vi "MainMeasure.vi"(8 "error in (no error)":errorcluster, 11 "TestMeasureStep in":refnum<class "TestMeasureStep.lvclass">) -> (0 "error out":errorcluster, 3 "TestMeasureStep out":refnum<class "TestMeasureStep.lvclass">)   [LabVIEW 2019, in "TestMeasureStep.lvclass"]
uses:
  TestMeasureStep.lvclass
  testSeq/Typedef/TestStatus.ctl
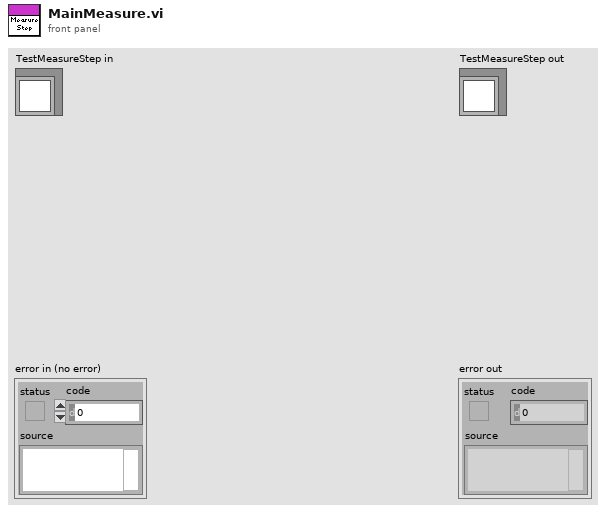
[diagram p1: front panel]
types:
  T1 = typedef "TestStatus.ctl" = enum16{"Not Executed", "Passed", "Failed", "Inconclusive", "Processing"}
  T2 = typedef "TestSeqClass.lvclass/TesstepType.ctl" = cluster{"TestName":string, "Meas":dbl, "Min ":dbl, "Max":dbl, "TestStatus":T1, "StringLimit":string, "StringMeas":string, "Unit":string}
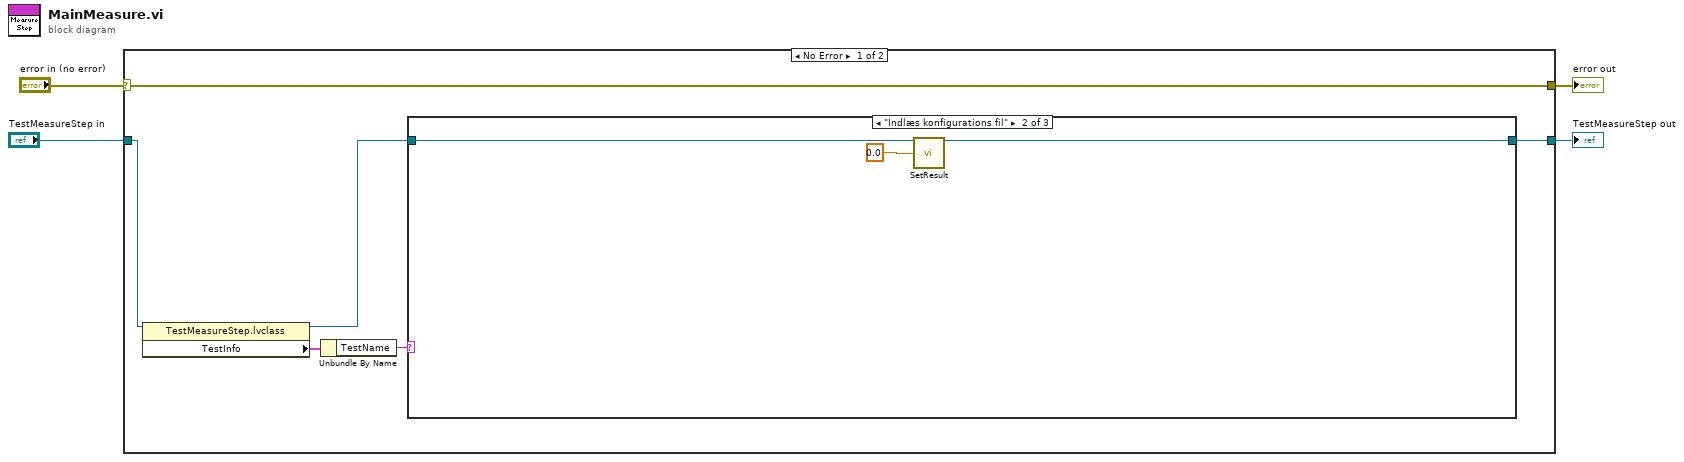
[diagram p0: block diagram]
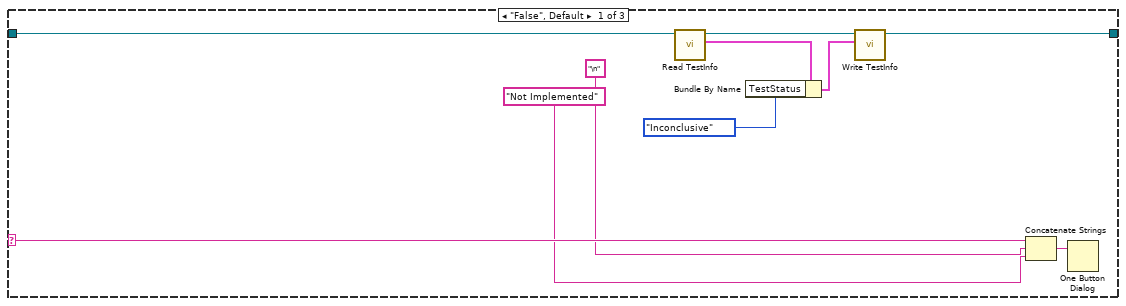
[diagram p2: hidden frame]
diagram:
  n1 = case shown="No Error" "error in (no error)" {
    selector: "error in (no error)" -> [w10 w26]
    tunnel: [w10 w26] -> w3
    tunnel: [w5 w25] -> w1
    tunnel: "TestMeasureStep in" -> [w9 w25]
    frame No Error {
      n2 = property class="TestMeasureStep.lvclass"(reference=w9) -> (reference out=w7:refnum<class "TestMeasureStep.lvclass">, "TestInfo"=w8:T2)  [unwired: 1 in, 1 out]
      n3 = Unbundle By Name(w8) -> ("TestName"=w6:string)
      n4 = case shown="\"Indlæs konfigurations fil\"" w6 {
        selector: w6 -> [w19 _ _]
        tunnel: w7 -> [w16 w23 w24]
        tunnel: [w11 w21 w24] -> w5
        frame "False", Default {
          n5 = call-dynamic "Read TestInfo.vi"("TestMeasureStep in"=w16) -> ("TestInfo 2"=w15:T2, "TestMeasureStep out"=w12:refnum<class "TestMeasureStep.lvclass">)  [unwired: 8 in, 1 out]
          n6 = Bundle By Name(cluster=w15, "TestStatus"=TestStatus."Inconclusive") -> (w13:T2)
          n7 = call-dynamic "Write TestInfo.vi"("TestInfo 2"=w13, "TestMeasureStep in"=w12) -> ("TestMeasureStep out"=w11:refnum<class "TestMeasureStep.lvclass">)  [unwired: 8 in, 1 out]
          n8 = Concatenate Strings(w19, "\n" ("string"), "Not Implemented" ("string")) -> (w20:string)
          n9 = One Button Dialog(message=w20) -> ()  [unwired: 1 in, 1 out]
        }
        frame "Indlæs konfigurations fil" {
          n10 = call "SetResult.vi"("TestMeasureStep in"=w23, "Meas"=0.0) -> ("TestMeasureStep out"=w21:refnum<class "TestMeasureStep.lvclass">)  [unwired: 11 in, 2 out]
        }
        frame "" {
        }
      }
    }
    frame Error {
    }
  }
  "error out" <- w3
  "TestMeasureStep out" <- w1
